vi "Launcher.vi"   [LabVIEW 2020]
uses:
  Generador/Generador.lvclass
  C:/Program Files (x86)/National Instruments/LabVIEW 2020/vi.lib/ActorFramework/Actor/Actor.lvclass
  <vilib>/ActorFramework/Actor/Actor.lvclass
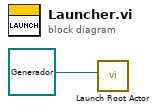
[diagram p0: block diagram]
diagram:
  n1 = call <vilib>:"Launch Root Actor.vi"("Actor"=refnum<class "Generador.lvclass"> refnum ("Generador.lvlib:Generador.lvclass")) -> ()  [unwired: 9 in, 2 out]
